vi "count rate.vi"() -> ()   [LabVIEW 2014]
uses:
  <vilib>/Platform/TimedLoop/XDataNode/timing_clust.ctl
  <vilib>/Platform/TimedLoop/XDataNode/nitl_modes.ctl
  <vilib>/Platform/TimedLoop/XDataNode/wakeup.ctl
  <vilib>/Utility/file.llb/Write To Spreadsheet File (I64).vi
  <vilib>/platform/TimedLoop/XDataNode/XDataNode.xnode
  <vilib>/Platform/TimedLoop/XDataNode/XDNodeRunTimeDep.lvlib
panel:
  out "Array":i64[](array[numeric])
  out "Array 2":dbl[](array[numeric])
  out "Waveform Graph":i32[](graph)
  in  "Total Time (sec)":dbl
  in  "Time Increment (msec)":i64=1000
  out "counts per second":dbl(knob) scale=0.0..100.0
  in  "stop":bool
  # "Demo count rate VI for Physics 434"
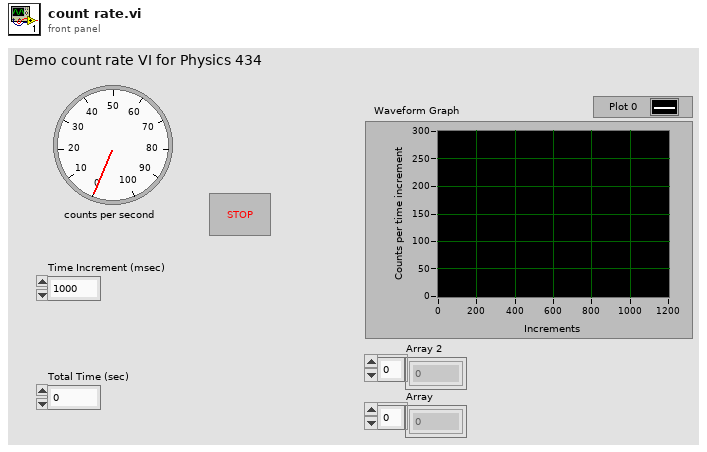
[diagram p1: front panel]
types:
  T1 = typedef "XDNodeRunTimeDep.lvlib/timing_clust.ctl" = cluster{"Expected End [f-1]":u64, "Actual End [f-1]":u64, "Finished Late? [f-1]":bool, "Expected End [i-1]":u64, "Actual End [i-1]":u64, "Finished Late? [i-1]":bool, "Expected Start [i]":u64, "Actual Start [i]":u64, "Expected Start [f]":u64, "Actual Start [f]":u64, "Source Name":string, "Structure Name":string, "Period":i64, "Deadline":i64, "Offset":i64, "Start":i64, "Priority":i32, "Timeout":i32, "Mode":T2, "Wakeup Reason":T3, "Error":errorcluster, "Source Type":string, "Secondary Source Type":string, "Global End Time":u64, "Global Start Time":u64, "Frame Duration":u64, "Iteration Duration":u64, "Assigned CPU":i32, "I/O Scan Engine Mode":u32}
  T2 = typedef "XDNodeRunTimeDep.lvlib/nitl_modes.ctl" = enum32{"No Change", "Process missed periods, maintain original phase", "Discard missed periods, maintain original phase", "Process missed periods, ignore original phase", "Discard missed periods, ignore original phase"}
  T3 = typedef "XDNodeRunTimeDep.lvlib/wakeup.ctl" = enum32{"Normal", "Aborted", "Asynchronous wakeup", "Timing source error", "Timed loop error", "Timeout"}
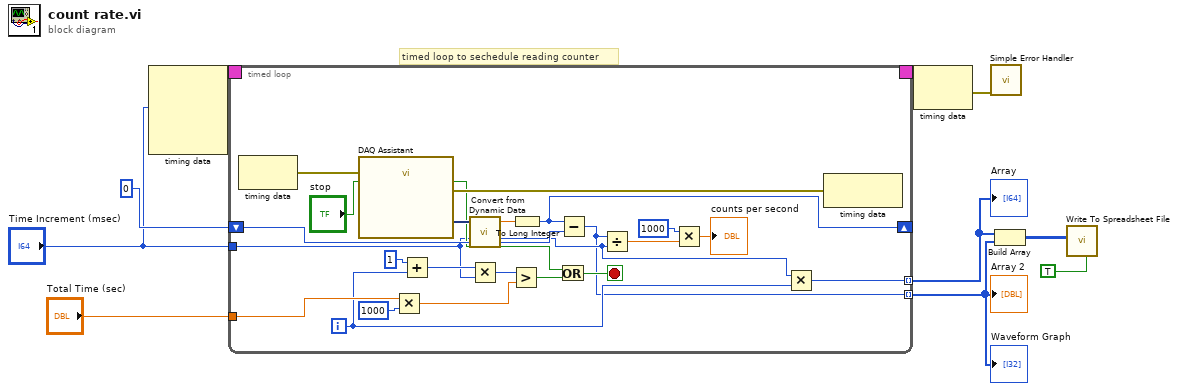
[diagram p0: block diagram]
diagram:
  # "timed loop to sechedule reading counter"
  n1 = node-c288("Time Increment (msec)") -> (w10:T1)  [unwired: 3 in]
  n2 = timed-loop {
    timing: w10 -> [_]
    timing-out: [_] -> w9
    shift-right: [w15] -> _
    shift-left: 0 -> [w32]
    tunnel: "Total Time (sec)" -> [w24]
    tunnel: "Time Increment (msec)" -> [w13]
    tunnel: [w11] -> w3 mode=indexing
    tunnel: [w12] -> w4 mode=indexing
    i -> [w14]
    stop <- w26 stop-if-true
    n3 = node-c288() -> (w28:errorcluster)  [unwired: 1 in]
    n4 = call "DAQ Assistant"("error in"=w28, "stop (F)"="stop") -> ("data"=w33:dynamicdata, "stopped"=w27:bool, "error out"=w29:errorcluster)  [unwired: 14 in, 1 out]
    n5 = Multiply(x=w24, y=1000) -> (x*y=w16:dbl)
    n6 = Add(x=1, y=w14) -> (x+y=w20:i32)
    n7 = call "Convert from Dynamic Data"("Dynamic Data Type"=w33) -> ("Scalar"=w30:dbl)  [unwired: 3 in]
    n8 = Multiply(x=w20, y=w13) -> (x*y=w17:i64)
    n9 = Greater?(x=w17, y=w16) -> (0:w18:bool)
    n10 = To Long Integer(number=w30) -> (32bit integer=w15:i32)
    n11 = Or(x=w27, y=w18) -> (x .or. y?=w26:bool)
    n12 = Subtract(x=w15, y=w32) -> (x-y=w11:i32)
    n13 = Divide(x=w11, y=w13) -> (x/y=w22:dbl)
    n14 = Multiply(x=1000, y=w22) -> (x*y=→"counts per second":dbl)
    n15 = Multiply(x=w13, y=w14) -> (x*y=w12:i64)
    n16 = node-c288(w29) -> ()  [unwired: 1 out]
  }
  "Waveform Graph" <- w3
  "Array 2" <- w3
  "Array" <- w4
  n17 = node-c288(w9) -> (w7:errorcluster)
  n18 = call <vilib>:"Simple Error Handler.vi"("error in (no error)"=w7) -> ()  [unwired: 4 in, 5 out]
  n19 = Build Array(w4, w3) -> (w2:i64[][])
  n20 = call-poly <vilib>:"Write To Spreadsheet File.vi"("transpose? (no:F)"=TRUE, "2D data"=w2) -> ()  [unwired: 6 in, 1 out]
